vi "_XNET Database Close All Except This.vi"(0 "database in":refnum<k21>, 11 "error in (no error)":errorcluster) -> (15 "error out":errorcluster)   [LabVIEW 2018]
doc: "Closes a database object (or all objects in the database)."
uses:
  nixlvapi.dll
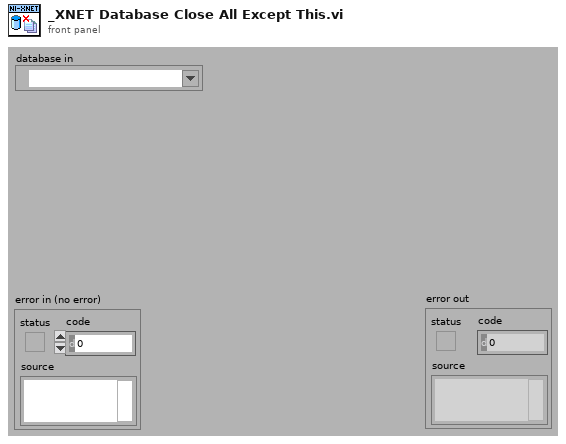
[diagram p1: front panel]
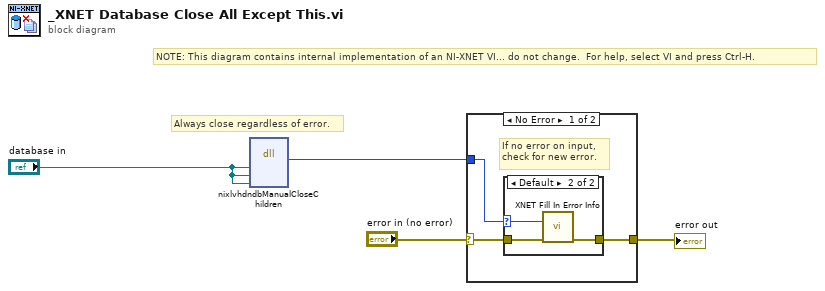
[diagram p0: block diagram]
diagram:
  # "Always close regardless of error."
  # "NOTE: This diagram contains internal implementation of an NI-XNET VI... do not change.  For help, select VI and press Ctrl-H."
  n1 = dll-call lib="nixlvapi.*" fn="nixlvhdndbManualCloseChildren"("reference"="database in", "lvObjectName"="database in", "refObjPtr"="database in") -> ("return type"=w1:i32)  [unwired: 4 in, 4 out]
  n2 = case shown="No Error" "error in (no error)" {
    selector: "error in (no error)" -> [w6 w12]
    tunnel: [w7 w12] -> w4
    tunnel: w1 -> [w5 _]
    frame No Error {
      # "If no error on input, \ncheck for new error."
      n3 = case shown="Default" w5 {
        selector: w5 -> [_ w9]
        tunnel: w6 -> [w8 w10]
        tunnel: [w8 w11] -> w7
        frame 0 {
        }
        frame Default {
          n4 = call "XNET Fill In Error Info.vi"("status code"=w9, "error in"=w10) -> ("error out"=w11:errorcluster)  [unwired: 13 out]
        }
      }
    }
    frame Error {
    }
  }
  "error out" <- w4
